vi "Variant to JSON.vi"(7 "Treatment of Infinity/NaN":T1, 8 "error in (no error)":errorcluster, 10 "Variant":variant) -> (0 "error out":errorcluster, 3 "JSON Value out":refnum<class "JSON Value.lvclass">)   [LabVIEW 2011, in "Variant JSON.lvlib"]
doc: "Converts a LabVIEW datatype (<b>Variant</b>) into a JSON value. Clusters are converted to JSON Objects. Variants, if empty (void), are converted to null, unless they have attributes, in which case these are converted into a JSON object. \n\nTreatment of Infinity, -Infinity, and Not-a-Number values of floating-point numerics:\n<b>-- Default JSON:</b> write all as nulls.\n<b>-- Extended:</b> use JSON strings for Infinities (\"Infinity\", \"-Infinity\"); NaN still null.\n<b>-- LabVIEW extentions</b> (compatable with the LabVIEW JSON primatives): Infinity, -Infinity, NaN (not in quotes)\n\nNote that the LabVIEW extentions are not valid JSON. The Extended option <b>is</b> valid JSON, but not all JSON parsers will process strings as numeric values.\n\nMore information on http://lavag.org/topic/16217-cr-json-labview"
uses:
  Variant JSON.lvlib
  JSON Value/JSON Value.lvclass
  JSON Scalar/Infinity&NaN.ctl
  <vilib>/Utility/VariantDataType/Type.ctl
  JSON Object/JSON Object.lvclass
  JSON Array/JSON Array.lvclass
  JSON Array/JSON Array.lvclass/JSON Array.ctl
  JSON Value/Set from JSON string.vi
  JSON Scalar/Set Null.vi
  JSON Scalar/Set I32.vi
  JSON Scalar/Set I64.vi
  JSON Scalar/Set U32.vi
  JSON Scalar/Set U64.vi
  JSON Scalar/Set SGL.vi
  JSON Scalar/Set EXT.vi
  JSON Scalar/Set Boolean.vi
  JSON Scalar/Set Path.vi
  JSON Scalar/Set Timestamp.vi
  JSON Scalar/JSON Scalar.lvclass
  Get Polymorphic/JSON GetSet.lvlib
  <vilib>/Utility/VariantDataType/VariantType.lvlib
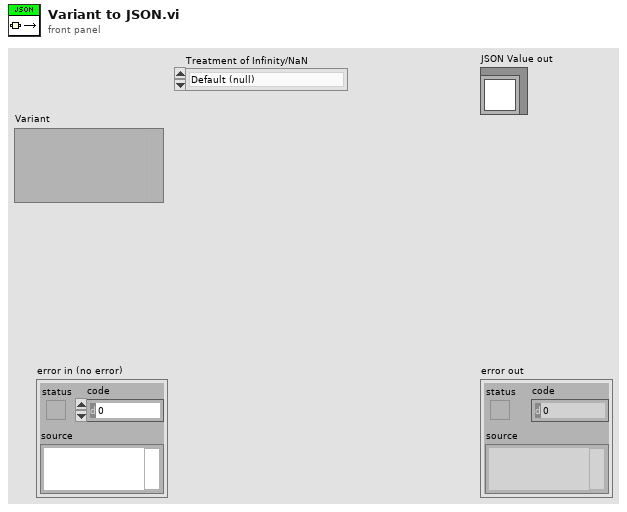
[diagram p1: front panel]
types:
  T1 = typedef "JSON Scalar.lvclass/Infinity&NaN.ctl" = enum16{"Default (null)", "Extended", "LabVIEW extensions"}
  T2 = typedef "VariantType.lvlib/Type.ctl" = enum8{"Invalid Type", "Void", "I8", "I16", "I32", "I64", "U8", "U16", "U32", "U64", "Single Float", "Double Float", "Extended Float", "Single Complex", "Double Complex", "Extended Complex", "Enum U8", "Enum U16", "Enum U32", "Enum U64", "Single Float With Unit", "Double Float With Unit", "Extended Float With Unit", "Single Complex with Unit", "Double Complex with Unit", "Extended Complex with Unit", "Boolean", "String", "Path", "Picture", "Tag", "Array", "Cluster", "Variant", "LV Variant", "Waveform", "Timestamp", "Digital Waveform", "Digital Data", "ExpressData", "Refnum", "External Data", "VI", "Poly VI", "LabVIEW Class Instance", "Fixed Point"}
  T3 = typedef "JSON Scalar.lvclass/Variant Data Typdef.ctl" = cluster{"Type Enum":T2, "Name":string, "Variant":variant}
  T4 = typedef "VariantType.lvlib/RefnumType.ctl" = enum16{"NotARefnum", "UnknownRefnum", "Generic", "Datalog", "ByteStream", "Device", "Occurence", "TCPNetConnection", "Auto", "Menu", "Imaq", "Hardware", "DataSocket", "Visa", "IVI", "UDPNetConnection", "Notifier", "Queue", "Irda", "EventReg", "DotNet", "UserEvent", "Callback", "UNUSED_EMPTY_POSITION", "BlueToothNetConnection", "LVObjApp", "LVObjVI", "LVObjUnknown", "GenericClass", "UserDefinedRefnumTag", "DataValue"}
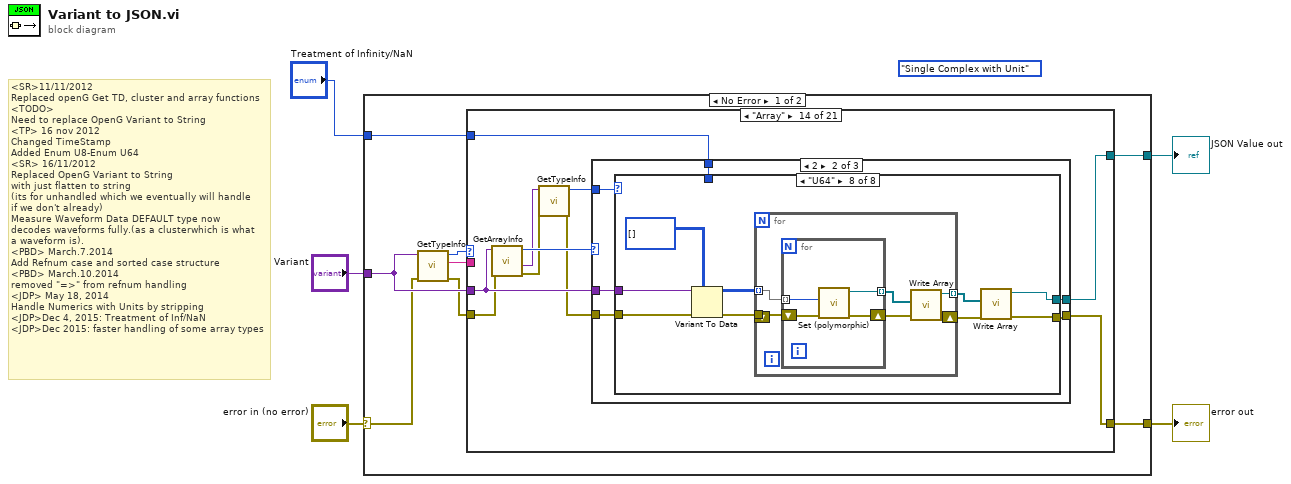
[diagram p0: block diagram]
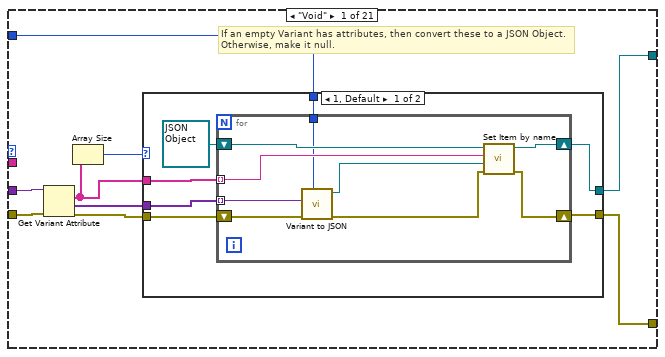
[diagram p2: hidden frame]
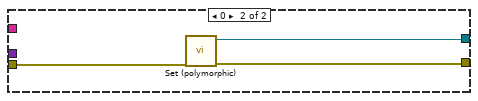
[diagram p3: hidden frame]
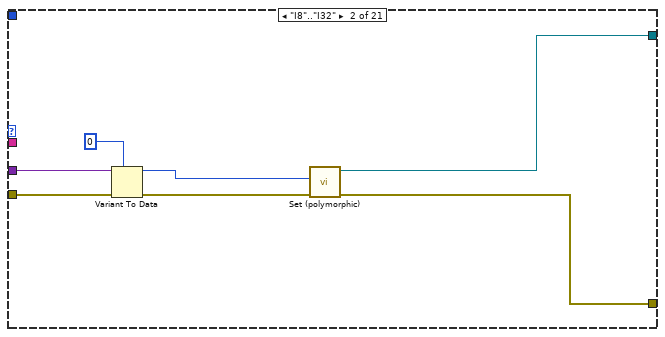
[diagram p4: hidden frame]
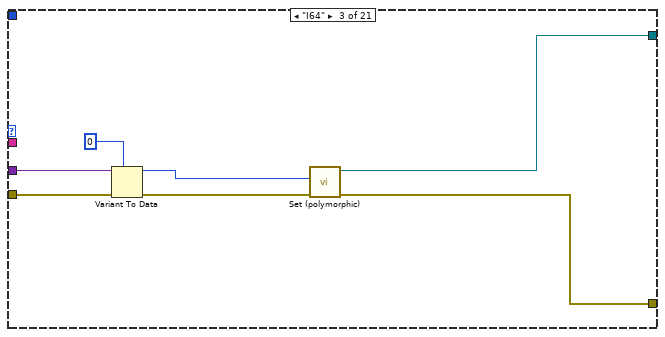
[diagram p5: hidden frame]
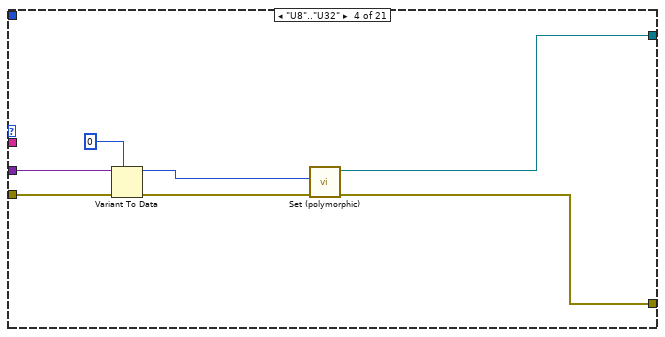
[diagram p6: hidden frame]
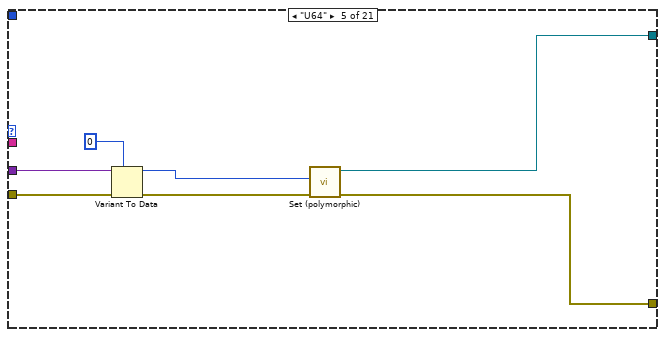
[diagram p7: hidden frame]
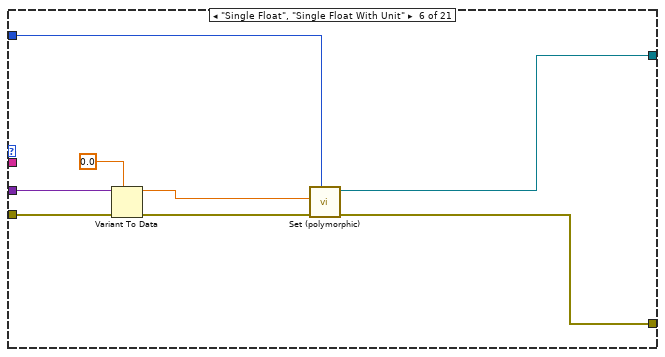
[diagram p8: hidden frame]
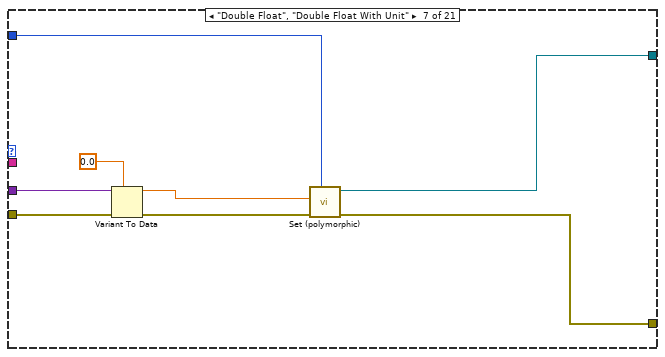
[diagram p9: hidden frame]
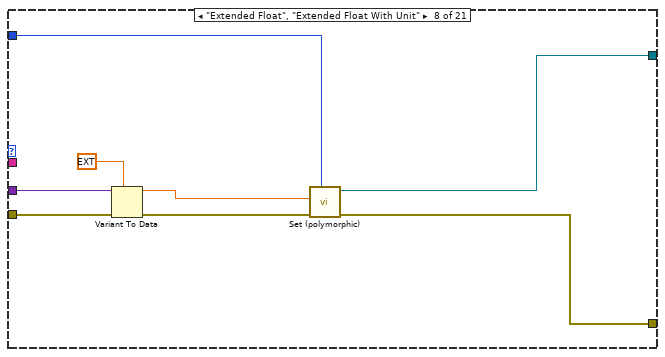
[diagram p10: hidden frame]
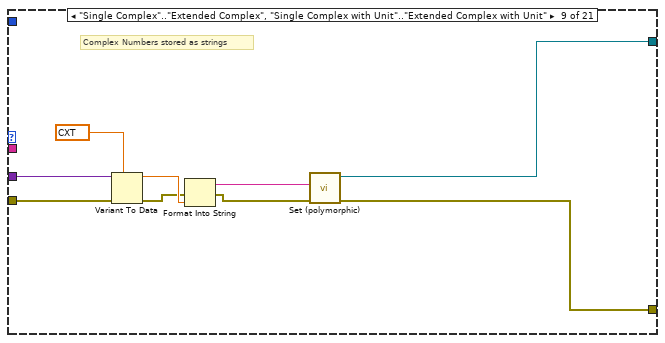
[diagram p11: hidden frame]
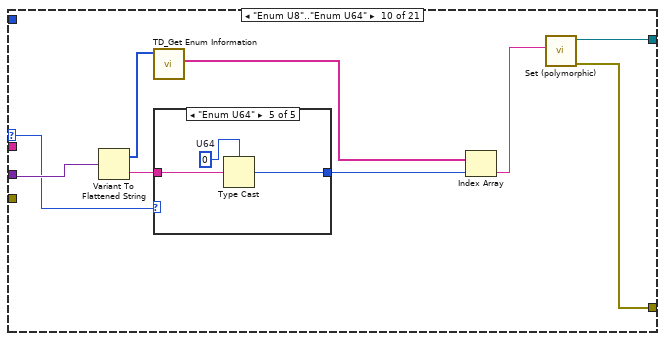
[diagram p12: hidden frame]
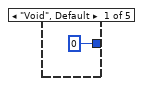
[diagram p13: hidden frame]
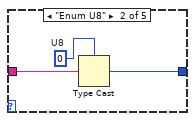
[diagram p14: hidden frame]
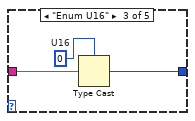
[diagram p15: hidden frame]
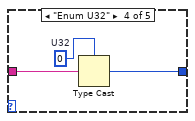
[diagram p16: hidden frame]
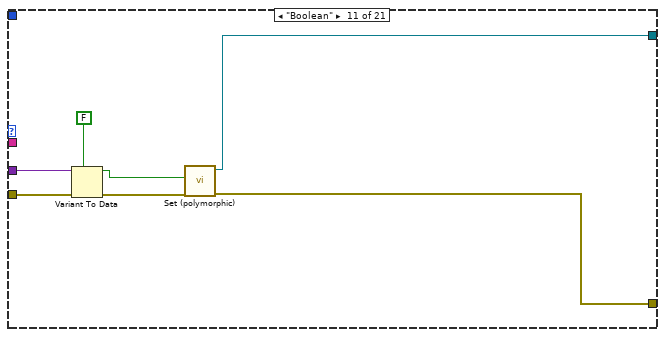
[diagram p17: hidden frame]
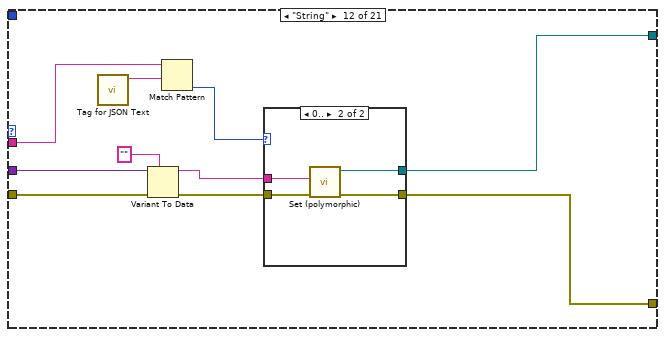
[diagram p18: hidden frame]
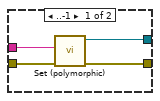
[diagram p19: hidden frame]
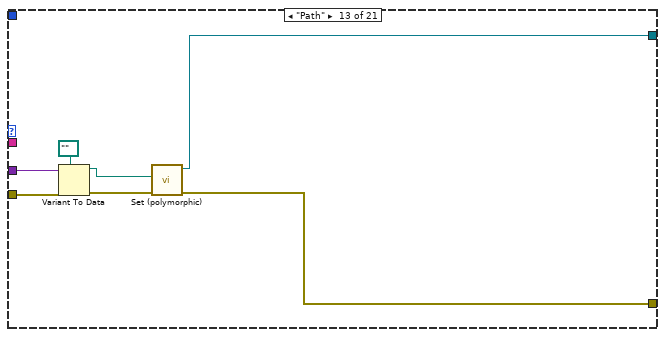
[diagram p20: hidden frame]
diagram:
  (unwired) Type."Single Complex with Unit" ("Type Enum")
  # "<SR>11/11/2012\nReplaced openG Get TD, cluster and array functions\n<TODO>\nNeed to replace OpenG Variant to String\n<TP> 16 nov 2012\nChanged TimeStamp\nAdded Enum U8-Enum U64\n<SR> 16/11/2012\nReplaced OpenG Variant to String\nwith just flatten to string \n(its for unhandled which we eventually will handle\nif we don't already)\nMeasure Waveform Data DEFAULT type now \ndecodes waveforms fully.(as a clusterwhich is what\na waveform is).\n<PBD> March.7.2014\nAdd Refnum case and sorted case structure\n<PBD> March.10.2014\nremoved \"=>\" from refnum handling\n<JDP> May 18, 2014\nHandle Numerics with Units by stripping\n<JDP>Dec 4, 2015: Treatment of Inf/NaN\n<JDP>Dec 2015: faster handling of some array types"
  n1 = case shown="No Error" "error in (no error)" {
    selector: "error in (no error)" -> [w10 w596]
    tunnel: [w12 w596] -> w4
    tunnel: [w13 _] -> w3
    tunnel: "Variant" -> [w11 _]
    tunnel: "Treatment of Infinity/NaN" -> [w6 _]
    frame No Error {
      n2 = call <vilib>:"GetTypeInfo.vi"("error in (no error)"=w10, "Variant"=w11) -> ("error out"=w9:errorcluster, "Name"=w7:string, "Type Enum"=w8:T2)  [unwired: 5 in, 2 out]
      n3 = case shown="\"Array\"" w8 {
        selector: w8 -> [_ _ _ _ _ _ _ _ _ w104 _ _ _ _ _ _ _ _ _ _ _]
        tunnel: w11 -> [w20 w48 w55 w62 w69 w77 w85 w93 w102 w105 w131 w141 w156 w163 w508 w526 w537 w544 w550 w580 w592]
        tunnel: [w22 w45 w52 w59 w66 w74 w82 w90 w101 w111 w128 w138 w152 w165 w511 w531 w539 w546 w548 w574 w595] -> w13
        tunnel: [w21 w43 w50 w57 w64 w72 w80 w88 w100 w110 w126 w136 w151 w166 w510 w530 w538 w545 w547 w573 w594] -> w12
        tunnel: w9 -> [w15 w42 w49 w56 w63 w71 w79 w87 w99 _ w125 w135 w154 w162 w506 w525 w536 w540 w549 w579 w593]
        tunnel: w7 -> [_ _ _ _ _ _ _ _ _ _ _ w133 _ _ _ _ _ _ _ _ _]
        tunnel: w6 -> [w14 _ _ _ _ w70 w78 w86 _ _ _ _ _ w164 w505 w524 w535 _ _ _ _]
        frame "Void" {
          # "If an empty Variant has attributes, then convert these to a JSON Object.\nOtherwise, make it null."
          n4 = Get Variant Attribute(Variant=w20, error in=w15) -> (names=w18:string[], values=w17:variant[], error out=w16:errorcluster)  [unwired: 2 in, 1 out]
          n5 = Array Size(array=w18) -> (size(s)=w19:i32)
          n6 = case shown="1, Default" w19 {
            tunnel: [w25 w40] -> w21
            tunnel: [w24 w41] -> w22
            tunnel: w18 -> [w27 _]
            tunnel: w17 -> [w29 _]
            tunnel: w16 -> [w28 w39]
            tunnel: w14 -> [w23 _]
            frame 1, Default {
              n7 = for {
                tunnel: w29 -> [w35] mode=indexing
                shift-right: [w31] -> w25
                shift-left: w28 -> [w34]
                tunnel: w27 -> [w36] mode=indexing
                shift-right: [w38] -> w24
                shift-left: refnum<class "JSON Object.lvclass"> refnum ("JSON Object out") -> [w37]
                tunnel: w23 -> [w30]
                n8 = call "Variant to JSON.vi"("Treatment of Infinity/NaN"=w30, "error in (no error)"=w34, "Variant"=w35) -> ("error out"=w32:errorcluster, "JSON Value out"=w33:refnum<class "JSON Value.lvclass">)  [unwired: 7 in]
                n9 = call-dynamic "Set Item by name.vi"("error in (no error)"=w32, "Value"=w33, "name"=w36, "JSON Object in"=w37) -> ("error out"=w31:errorcluster, "JSON Object out"=w38:refnum<class "JSON Object.lvclass">)  [unwired: 5 in, 1 out]
              }
            }
            frame 0 {
              n10 = call-poly "Set (polymorphic).vi"("error in (no error)"=w39) -> ("error out"=w40:errorcluster, "JSON Scalar out"=w41:refnum<class "JSON Scalar.lvclass">)  [unwired: 9 in]
            }
          }
        }
        frame "I8".."I32" {
          n11 = Variant To Data(error in=w42, type=0, Variant=w48) -> (data=w46:i32, error out=w44:errorcluster)
          n12 = call-poly "Set (polymorphic).vi"("error in (no error)"=w44, "Numeric"=w46) -> ("error out"=w43:errorcluster, "JSON Scalar out"=w45:refnum<class "JSON Scalar.lvclass">)  [unwired: 8 in]
        }
        frame "I64" {
          n13 = Variant To Data(error in=w49, type=i64 0, Variant=w55) -> (data=w53:i64, error out=w51:errorcluster)
          n14 = call-poly "Set (polymorphic).vi"("error in (no error)"=w51, "Numeric"=w53) -> ("error out"=w50:errorcluster, "JSON Scalar out"=w52:refnum<class "JSON Scalar.lvclass">)  [unwired: 8 in]
        }
        frame "U8".."U32" {
          n15 = Variant To Data(error in=w56, type=u32 0, Variant=w62) -> (data=w60:u32, error out=w58:errorcluster)
          n16 = call-poly "Set (polymorphic).vi"("error in (no error)"=w58, "Numeric"=w60) -> ("error out"=w57:errorcluster, "JSON Scalar out"=w59:refnum<class "JSON Scalar.lvclass">)  [unwired: 8 in]
        }
        frame "U64" {
          n17 = Variant To Data(error in=w63, type=u64 0, Variant=w69) -> (data=w67:u64, error out=w65:errorcluster)
          n18 = call-poly "Set (polymorphic).vi"("error in (no error)"=w65, "Numeric"=w67) -> ("error out"=w64:errorcluster, "JSON Scalar out"=w66:refnum<class "JSON Scalar.lvclass">)  [unwired: 8 in]
        }
        frame "Single Float", "Single Float With Unit" {
          n19 = Variant To Data(error in=w71, type=sgl 0.0, Variant=w77) -> (data=w75:sgl, error out=w73:errorcluster)
          n20 = call-poly "Set (polymorphic).vi"("Treatment of Infinity/NaN"=w70, "error in (no error)"=w73, "Numeric"=w75) -> ("error out"=w72:errorcluster, "JSON Scalar out"=w74:refnum<class "JSON Scalar.lvclass">)  [unwired: 7 in]
        }
        frame "Double Float", "Double Float With Unit" {
          n21 = Variant To Data(error in=w79, type=0.0, Variant=w85) -> (data=w83:dbl, error out=w81:errorcluster)
          n22 = call-poly "Set (polymorphic).vi"("Treatment of Infinity/NaN"=w78, "error in (no error)"=w81, "Numeric"=w83) -> ("error out"=w80:errorcluster, "JSON Scalar out"=w82:refnum<class "JSON Scalar.lvclass">)  [unwired: 7 in]
        }
        frame "Extended Float", "Extended Float With Unit" {
          n23 = Variant To Data(error in=w87, type=ext 0.0, Variant=w93) -> (data=w91:ext, error out=w89:errorcluster)
          n24 = call-poly "Set (polymorphic).vi"("Treatment of Infinity/NaN"=w86, "error in (no error)"=w89, "Numeric"=w91) -> ("error out"=w88:errorcluster, "JSON Scalar out"=w90:refnum<class "JSON Scalar.lvclass">)  [unwired: 7 in]
        }
        frame "Single Complex".."Extended Complex", "Single Complex with Unit".."Extended Complex with Unit" {
          # "Complex Numbers stored as strings"
          n25 = Variant To Data(error in=w99, type=cxt 0.0+0.0i, Variant=w102) -> (data=w97:cxt, error out=w95:errorcluster)
          n26 = Format Into String(error in=w95, w97) -> (resulting string=w96:string, error out=w94:errorcluster)  [unwired: 2 in]
          n27 = call-poly "Set (polymorphic).vi"("error in (no error)"=w94, "String"=w96) -> ("error out"=w100:errorcluster, "JSON Scalar out"=w101:refnum<class "JSON Scalar.lvclass">)  [unwired: 8 in]
        }
        frame "Enum U8".."Enum U64" {
          n28 = Variant To Flattened String(Variant=w105) -> (data string=w108:string, 1:w109:i16[])
          n29 = call <vilib>:"TD_Get Enum Information.vi"("Type descriptor"=w109) -> ("Value Names"=w107:string[])  [unwired: 9 in, 1 out]
          n30 = case shown="\"Enum U64\"" w104 {
            tunnel: w108 -> [_ w115 w118 w121 w124]
            tunnel: [u64 0 ("U8") w113 w116 w119 w122] -> w106
            frame "Void", Default {
            }
            frame "Enum U8" {
              w114 = u8 0  # U8
              n31 = Type Cast(type=w114, x=w115) -> (*(type *) &x=w113:u8)
            }
            frame "Enum U16" {
              w117 = u16 0  # U16
              n32 = Type Cast(type=w117, x=w118) -> (*(type *) &x=w116:u16)
            }
            frame "Enum U32" {
              w120 = u32 0  # U32
              n33 = Type Cast(type=w120, x=w121) -> (*(type *) &x=w119:u32)
            }
            frame "Enum U64" {
              w123 = u64 0  # U64
              n34 = Type Cast(type=w123, x=w124) -> (*(type *) &x=w122:u64)
            }
          }
          n35 = Index Array(array=w107, index=w106) -> (element=w103:string)
          n36 = call-poly "Set (polymorphic).vi"("String"=w103) -> ("error out"=w110:errorcluster, "JSON Scalar out"=w111:refnum<class "JSON Scalar.lvclass">)  [unwired: 9 in]
        }
        frame "Boolean" {
          n37 = Variant To Data(error in=w125, type=FALSE, Variant=w131) -> (data=w129:bool, error out=w127:errorcluster)
          n38 = call-poly "Set (polymorphic).vi"("error in (no error)"=w127, "Boolean"=w129) -> ("error out"=w126:errorcluster, "JSON Scalar out"=w128:refnum<class "JSON Scalar.lvclass">)  [unwired: 8 in]
        }
        frame "String" {
          n39 = call "Tag for JSON Text.vi"() -> ("Tag for JSON text"=w134:string)  [unwired: 11 in]
          n40 = Variant To Data(error in=w135, type="", Variant=w141) -> (data=w139:string, error out=w137:errorcluster)
          n41 = Match Pattern(string=w133, regular expression=w134) -> (offset past match=w132:i32)  [unwired: 1 in, 3 out]
          n42 = case shown="0.." w132 {
            tunnel: w139 -> [w145 w149]
            tunnel: [w144 w148] -> w138
            tunnel: w137 -> [w143 w147]
            tunnel: [w142 w146] -> w136
            frame ..-1 {
              n43 = call-poly "Set (polymorphic).vi"("error in (no error)"=w143, "String"=w145) -> ("error out"=w142:errorcluster, "JSON Scalar out"=w144:refnum<class "JSON Scalar.lvclass">)  [unwired: 8 in]
            }
            frame 0.. {
              n44 = call-poly "Set (polymorphic).vi"("error in (no error)"=w147, "JSON stream"=w149) -> ("error out"=w146:errorcluster, "JSON Value out"=w148:refnum<class "JSON Value.lvclass">)  [unwired: 7 in, 1 out]
            }
          }
        }
        frame "Path" {
          n45 = Variant To Data(error in=w154, type=path "", Variant=w156) -> (data=w150:path, error out=w153:errorcluster)
          n46 = call-poly "Set (polymorphic).vi"("error in (no error)"=w153, "Path"=w150) -> ("error out"=w151:errorcluster, "JSON Scalar out"=w152:refnum<class "JSON Scalar.lvclass">)  [unwired: 8 in]
        }
        frame "Array" {
          n47 = call <vilib>:"GetArrayInfo.vi"("error in (no error)"=w162, "Variant"=w163) -> ("error out"=w160:errorcluster, "ArrayElement"=w159:variant, "NDims"=w161:i32)  [unwired: 6 in, 1 out]
          n48 = call <vilib>:"GetTypeInfo.vi"("error in (no error)"=w160, "Variant"=w159) -> ("error out"=w158:errorcluster, "Type Enum"=w157:T2)  [unwired: 5 in, 3 out]
          n49 = case shown="2" w161 {
            tunnel: [w171 w331 w504] -> w166
            tunnel: [w170 w330 w500] -> w165
            tunnel: w164 -> [w168 w328 w499]
            tunnel: w163 -> [w172 w332 w498]
            tunnel: w158 -> [w169 w329 w497]
            tunnel: w157 -> [w167 w327 _]
            frame 1 {
              n50 = case shown="\"Waveform\"" w167 {
                tunnel: w172 -> [w183 w197 w211 w226 w241 w255 w268 w281 w294 w307 w321]
                tunnel: [w177 w191 w205 w220 w235 w249 w262 w275 w288 w301 w315] -> w171
                tunnel: [w176 w190 w204 w219 w234 w248 w261 w274 w287 w300 w314] -> w170
                tunnel: w169 -> [w174 w189 w203 w218 w233 w247 w260 w273 w286 w299 w313]
                tunnel: w168 -> [w173 _ w202 w217 w232 _ _ _ _ _ w312]
                frame Default {
                  n51 = Variant To Data(error in=w174, type=variant[] [], Variant=w183) -> (data=w181:variant[], error out=w180:errorcluster)
                  n52 = for {
                    tunnel: w181 -> [w188] mode=indexing
                    shift-right: [w186] -> w178
                    shift-left: w180 -> [w187]
                    tunnel: [w185] -> w179 mode=indexing
                    tunnel: w173 -> [w184]
                    n53 = call "Variant to JSON.vi"("Treatment of Infinity/NaN"=w184, "error in (no error)"=w187, "Variant"=w188) -> ("error out"=w186:errorcluster, "JSON Value out"=w185:refnum<class "JSON Value.lvclass">)  [unwired: 7 in]
                  }
                  n54 = call "Write Array.vi"("error in (no error)"=w178, "Array"=w179, "JSON Array in"=refnum<class "JSON Array.lvclass"> refnum) -> ("error out"=w177:errorcluster, "JSON Array out"=w176:refnum<class "JSON Array.lvclass">)  [unwired: 7 in]
                }
                frame "String" {
                  n55 = Variant To Data(error in=w189, type=string[] [], Variant=w197) -> (data=w195:string[], error out=w194:errorcluster)
                  n56 = for {
                    tunnel: w195 -> [w198] mode=indexing
                    shift-right: [w200] -> w192
                    shift-left: w194 -> [w201]
                    tunnel: [w199] -> w193 mode=indexing
                    n57 = call "Set String.vi"("error in (no error)"=w201, "String"=w198) -> ("error out"=w200:errorcluster, "JSON Scalar out"=w199:refnum<class "JSON Scalar.lvclass">)  [unwired: 8 in]
                  }
                  n58 = call "Write Array.vi"("error in (no error)"=w192, "Array"=w193) -> ("error out"=w191:errorcluster, "JSON Array out"=w190:refnum<class "JSON Array.lvclass">)  [unwired: 8 in]
                }
                frame "Single Float" {
                  n59 = Variant To Data(error in=w203, type=sgl[] [], Variant=w211) -> (data=w209:sgl[], error out=w208:errorcluster)
                  n60 = for {
                    tunnel: w209 -> [w212] mode=indexing
                    shift-right: [w215] -> w206
                    shift-left: w208 -> [w216]
                    tunnel: [w214] -> w207 mode=indexing
                    tunnel: w202 -> [w213]
                    n61 = call "Set DBL.vi"("Treatment of Infinity/NaN"=w213, "error in (no error)"=w216, "Numeric"=w212) -> ("error out"=w215:errorcluster, "JSON Scalar out"=w214:refnum<class "JSON Scalar.lvclass">)  [unwired: 7 in]
                  }
                  n62 = call "Write Array.vi"("error in (no error)"=w206, "Array"=w207) -> ("error out"=w205:errorcluster, "JSON Array out"=w204:refnum<class "JSON Array.lvclass">)  [unwired: 8 in]
                }
                frame "Double Float" {
                  n63 = Variant To Data(error in=w218, type=dbl[] [], Variant=w226) -> (data=w224:dbl[], error out=w223:errorcluster)
                  n64 = for {
                    tunnel: w224 -> [w227] mode=indexing
                    shift-right: [w230] -> w221
                    shift-left: w223 -> [w231]
                    tunnel: [w229] -> w222 mode=indexing
                    tunnel: w217 -> [w228]
                    n65 = call-poly "Set (polymorphic).vi"("Treatment of Infinity/NaN"=w228, "error in (no error)"=w231, "Numeric"=w227) -> ("error out"=w230:errorcluster, "JSON Scalar out"=w229:refnum<class "JSON Scalar.lvclass">)  [unwired: 7 in]
                  }
                  n66 = call "Write Array.vi"("error in (no error)"=w221, "Array"=w222) -> ("error out"=w220:errorcluster, "JSON Array out"=w219:refnum<class "JSON Array.lvclass">)  [unwired: 8 in]
                }
                frame "Extended Float" {
                  n67 = Variant To Data(error in=w233, type=ext[] [], Variant=w241) -> (data=w239:ext[], error out=w238:errorcluster)
                  n68 = for {
                    tunnel: w239 -> [w242] mode=indexing
                    shift-right: [w245] -> w236
                    shift-left: w238 -> [w246]
                    tunnel: [w244] -> w237 mode=indexing
                    tunnel: w232 -> [w243]
                    n69 = call-poly "Set (polymorphic).vi"("Treatment of Infinity/NaN"=w243, "error in (no error)"=w246, "Numeric"=w242) -> ("error out"=w245:errorcluster, "JSON Scalar out"=w244:refnum<class "JSON Scalar.lvclass">)  [unwired: 7 in]
                  }
                  n70 = call "Write Array.vi"("error in (no error)"=w236, "Array"=w237) -> ("error out"=w235:errorcluster, "JSON Array out"=w234:refnum<class "JSON Array.lvclass">)  [unwired: 8 in]
                }
                frame "I8".."I32" {
                  n71 = Variant To Data(error in=w247, type=i32[] [], Variant=w255) -> (data=w253:i32[], error out=w252:errorcluster)
                  n72 = for {
                    tunnel: w253 -> [w256] mode=indexing
                    shift-right: [w258] -> w250
                    shift-left: w252 -> [w259]
                    tunnel: [w257] -> w251 mode=indexing
                    n73 = call-poly "Set (polymorphic).vi"("error in (no error)"=w259, "Numeric"=w256) -> ("error out"=w258:errorcluster, "JSON Scalar out"=w257:refnum<class "JSON Scalar.lvclass">)  [unwired: 8 in]
                  }
                  n74 = call "Write Array.vi"("error in (no error)"=w250, "Array"=w251) -> ("error out"=w249:errorcluster, "JSON Array out"=w248:refnum<class "JSON Array.lvclass">)  [unwired: 8 in]
                }
                frame "I64" {
                  n75 = Variant To Data(error in=w260, type=i64[] [], Variant=w268) -> (data=w266:i64[], error out=w265:errorcluster)
                  n76 = for {
                    tunnel: w266 -> [w269] mode=indexing
                    shift-right: [w271] -> w263
                    shift-left: w265 -> [w272]
                    tunnel: [w270] -> w264 mode=indexing
                    n77 = call-poly "Set (polymorphic).vi"("error in (no error)"=w272, "Numeric"=w269) -> ("error out"=w271:errorcluster, "JSON Scalar out"=w270:refnum<class "JSON Scalar.lvclass">)  [unwired: 8 in]
                  }
                  n78 = call "Write Array.vi"("error in (no error)"=w263, "Array"=w264) -> ("error out"=w262:errorcluster, "JSON Array out"=w261:refnum<class "JSON Array.lvclass">)  [unwired: 8 in]
                }
                frame "U8".."U32" {
                  n79 = Variant To Data(error in=w273, type=u32[] [], Variant=w281) -> (data=w279:u32[], error out=w278:errorcluster)
                  n80 = for {
                    tunnel: w279 -> [w282] mode=indexing
                    shift-right: [w284] -> w276
                    shift-left: w278 -> [w285]
                    tunnel: [w283] -> w277 mode=indexing
                    n81 = call-poly "Set (polymorphic).vi"("error in (no error)"=w285, "Numeric"=w282) -> ("error out"=w284:errorcluster, "JSON Scalar out"=w283:refnum<class "JSON Scalar.lvclass">)  [unwired: 8 in]
                  }
                  n82 = call "Write Array.vi"("error in (no error)"=w276, "Array"=w277) -> ("error out"=w275:errorcluster, "JSON Array out"=w274:refnum<class "JSON Array.lvclass">)  [unwired: 8 in]
                }
                frame "U64" {
                  n83 = Variant To Data(error in=w286, type=u64[] [], Variant=w294) -> (data=w292:u64[], error out=w291:errorcluster)
                  n84 = for {
                    tunnel: w292 -> [w295] mode=indexing
                    shift-right: [w297] -> w289
                    shift-left: w291 -> [w298]
                    tunnel: [w296] -> w290 mode=indexing
                    n85 = call-poly "Set (polymorphic).vi"("error in (no error)"=w298, "Numeric"=w295) -> ("error out"=w297:errorcluster, "JSON Scalar out"=w296:refnum<class "JSON Scalar.lvclass">)  [unwired: 8 in]
                  }
                  n86 = call "Write Array.vi"("error in (no error)"=w289, "Array"=w290) -> ("error out"=w288:errorcluster, "JSON Array out"=w287:refnum<class "JSON Array.lvclass">)  [unwired: 8 in]
                }
                frame "Timestamp" {
                  n87 = Variant To Data(error in=w299, type=timestamp[] [], Variant=w307) -> (data=w305:timestamp[], error out=w304:errorcluster)
                  n88 = for {
                    tunnel: w305 -> [w308] mode=indexing
                    shift-right: [w310] -> w302
                    shift-left: w304 -> [w311]
                    tunnel: [w309] -> w303 mode=indexing
                    n89 = call-poly "Set (polymorphic).vi"("error in (no error)"=w311, "Time Stamp"=w308) -> ("error out"=w310:errorcluster, "JSON Scalar out"=w309:refnum<class "JSON Scalar.lvclass">)  [unwired: 8 in]
                  }
                  n90 = call "Write Array.vi"("error in (no error)"=w302, "Array"=w303) -> ("error out"=w301:errorcluster, "JSON Array out"=w300:refnum<class "JSON Array.lvclass">)  [unwired: 8 in]
                }
                frame "Waveform" {
                  n91 = Variant To Data(error in=w313, type=waveform(dbl)[] [], Variant=w321) -> (data=w319:waveform(dbl)[], error out=w318:errorcluster)
                  n92 = for {
                    tunnel: w319 -> [w323] mode=indexing
                    shift-right: [w325] -> w316
                    shift-left: w318 -> [w326]
                    tunnel: [w324] -> w317 mode=indexing
                    tunnel: w312 -> [w322]
                    n93 = call-poly "Set (polymorphic).vi"("Treatment of Infinity/NaN"=w322, "error in (no error)"=w326, "waveform"=w323) -> ("error out"=w325:errorcluster, "JSON Object out"=w324:refnum<class "JSON Object.lvclass">)  [unwired: 7 in]
                  }
                  n94 = call "Write Array.vi"("error in (no error)"=w316, "Array"=w317) -> ("error out"=w315:errorcluster, "JSON Array out"=w314:refnum<class "JSON Array.lvclass">)  [unwired: 8 in]
                }
              }
            }
            frame 2 {
              n95 = case shown="\"U64\"" w327 {
                tunnel: w332 -> [w342 w364 w386 w408 w429 w448 w467 w486]
                tunnel: [w334 w356 w378 w400 w422 w441 w460 w479] -> w331
                tunnel: [w333 w355 w377 w399 w421 w440 w459 w478] -> w330
                tunnel: w329 -> [w338 w360 w382 w404 w425 w444 w463 w482]
                tunnel: w328 -> [w337 w359 w381 w403 _ _ _ _]
                frame Default {
                  n96 = Variant To Data(error in=w338, type=variant[][] [], Variant=w342) -> (data=w340:variant[][], error out=w339:errorcluster)
                  n97 = for {
                    tunnel: w340 -> [w349] mode=indexing
                    tunnel: w339 -> [w348]
                    tunnel: [w344] -> w336 mode=indexing
                    tunnel: w337 -> [w343]
                    shift-right: [w345] -> w335
                    shift-left: _ -> [_]
                    n98 = for {
                      tunnel: w349 -> [w354] mode=indexing
                      shift-right: [w352] -> w346
                      shift-left: w348 -> [w353]
                      tunnel: [w351] -> w347 mode=indexing
                      tunnel: w343 -> [w350]
                      n99 = call "Variant to JSON.vi"("Treatment of Infinity/NaN"=w350, "error in (no error)"=w353, "Variant"=w354) -> ("error out"=w352:errorcluster, "JSON Value out"=w351:refnum<class "JSON Value.lvclass">)  [unwired: 7 in]
                    }
                    n100 = call "Write Array.vi"("error in (no error)"=w346, "Array"=w347) -> ("error out"=w345:errorcluster, "JSON Array out"=w344:refnum<class "JSON Array.lvclass">)  [unwired: 8 in]
                  }
                  n101 = call "Write Array.vi"("error in (no error)"=w335, "Array"=w336) -> ("error out"=w334:errorcluster, "JSON Array out"=w333:refnum<class "JSON Array.lvclass">)  [unwired: 8 in]
                }
                frame "Double Float" {
                  n102 = Variant To Data(error in=w360, type=dbl[][] [], Variant=w364) -> (data=w362:dbl[][], error out=w361:errorcluster)
                  n103 = for {
                    tunnel: w362 -> [w371] mode=indexing
                    tunnel: w361 -> [w370]
                    tunnel: [w366] -> w358 mode=indexing
                    tunnel: w359 -> [w365]
                    shift-right: [w367] -> w357
                    shift-left: _ -> [_]
                    n104 = for {
                      tunnel: w371 -> [w372] mode=indexing
                      shift-right: [w375] -> w368
                      shift-left: w370 -> [w376]
                      tunnel: [w374] -> w369 mode=indexing
                      tunnel: w365 -> [w373]
                      n105 = call "Set DBL.vi"("Treatment of Infinity/NaN"=w373, "error in (no error)"=w376, "Numeric"=w372) -> ("error out"=w375:errorcluster, "JSON Scalar out"=w374:refnum<class "JSON Scalar.lvclass">)  [unwired: 7 in]
                    }
                    n106 = call "Write Array.vi"("error in (no error)"=w368, "Array"=w369) -> ("error out"=w367:errorcluster, "JSON Array out"=w366:refnum<class "JSON Array.lvclass">)  [unwired: 8 in]
                  }
                  n107 = call "Write Array.vi"("error in (no error)"=w357, "Array"=w358) -> ("error out"=w356:errorcluster, "JSON Array out"=w355:refnum<class "JSON Array.lvclass">)  [unwired: 8 in]
                }
                frame "Single Float" {
                  n108 = Variant To Data(error in=w382, type=sgl[][] [], Variant=w386) -> (data=w384:sgl[][], error out=w383:errorcluster)
                  n109 = for {
                    tunnel: w384 -> [w393] mode=indexing
                    tunnel: w383 -> [w392]
                    tunnel: [w388] -> w380 mode=indexing
                    tunnel: w381 -> [w387]
                    shift-right: [w389] -> w379
                    shift-left: _ -> [_]
                    n110 = for {
                      tunnel: w393 -> [w394] mode=indexing
                      shift-right: [w397] -> w390
                      shift-left: w392 -> [w398]
                      tunnel: [w396] -> w391 mode=indexing
                      tunnel: w387 -> [w395]
                      n111 = call-poly "Set (polymorphic).vi"("Treatment of Infinity/NaN"=w395, "error in (no error)"=w398, "Numeric"=w394) -> ("error out"=w397:errorcluster, "JSON Scalar out"=w396:refnum<class "JSON Scalar.lvclass">)  [unwired: 7 in]
                    }
                    n112 = call "Write Array.vi"("error in (no error)"=w390, "Array"=w391) -> ("error out"=w389:errorcluster, "JSON Array out"=w388:refnum<class "JSON Array.lvclass">)  [unwired: 8 in]
                  }
                  n113 = call "Write Array.vi"("error in (no error)"=w379, "Array"=w380) -> ("error out"=w378:errorcluster, "JSON Array out"=w377:refnum<class "JSON Array.lvclass">)  [unwired: 8 in]
                }
                frame "Extended Float" {
                  n114 = Variant To Data(error in=w404, type=ext[][] [], Variant=w408) -> (data=w406:ext[][], error out=w405:errorcluster)
                  n115 = for {
                    tunnel: w406 -> [w415] mode=indexing
                    tunnel: w405 -> [w414]
                    tunnel: [w410] -> w402 mode=indexing
                    tunnel: w403 -> [w409]
                    shift-right: [w411] -> w401
                    shift-left: _ -> [_]
                    n116 = for {
                      tunnel: w415 -> [w416] mode=indexing
                      shift-right: [w419] -> w412
                      shift-left: w414 -> [w420]
                      tunnel: [w418] -> w413 mode=indexing
                      tunnel: w409 -> [w417]
                      n117 = call-poly "Set (polymorphic).vi"("Treatment of Infinity/NaN"=w417, "error in (no error)"=w420, "Numeric"=w416) -> ("error out"=w419:errorcluster, "JSON Scalar out"=w418:refnum<class "JSON Scalar.lvclass">)  [unwired: 7 in]
                    }
                    n118 = call "Write Array.vi"("error in (no error)"=w412, "Array"=w413) -> ("error out"=w411:errorcluster, "JSON Array out"=w410:refnum<class "JSON Array.lvclass">)  [unwired: 8 in]
                  }
                  n119 = call "Write Array.vi"("error in (no error)"=w401, "Array"=w402) -> ("error out"=w400:errorcluster, "JSON Array out"=w399:refnum<class "JSON Array.lvclass">)  [unwired: 8 in]
                }
                frame "I8".."I32" {
                  n120 = Variant To Data(error in=w425, type=i32[][] [], Variant=w429) -> (data=w427:i32[][], error out=w426:errorcluster)
                  n121 = for {
                    tunnel: w427 -> [w435] mode=indexing
                    tunnel: w426 -> [w434]
                    tunnel: [w430] -> w424 mode=indexing
                    shift-right: [w431] -> w423
                    shift-left: _ -> [_]
                    n122 = for {
                      tunnel: w435 -> [w436] mode=indexing
                      shift-right: [w438] -> w432
                      shift-left: w434 -> [w439]
                      tunnel: [w437] -> w433 mode=indexing
                      n123 = call-poly "Set (polymorphic).vi"("error in (no error)"=w439, "Numeric"=w436) -> ("error out"=w438:errorcluster, "JSON Scalar out"=w437:refnum<class "JSON Scalar.lvclass">)  [unwired: 8 in]
                    }
                    n124 = call "Write Array.vi"("error in (no error)"=w432, "Array"=w433) -> ("error out"=w431:errorcluster, "JSON Array out"=w430:refnum<class "JSON Array.lvclass">)  [unwired: 8 in]
                  }
                  n125 = call "Write Array.vi"("error in (no error)"=w423, "Array"=w424) -> ("error out"=w422:errorcluster, "JSON Array out"=w421:refnum<class "JSON Array.lvclass">)  [unwired: 8 in]
                }
                frame "I64" {
                  n126 = Variant To Data(error in=w444, type=i64[][] [], Variant=w448) -> (data=w446:i64[][], error out=w445:errorcluster)
                  n127 = for {
                    tunnel: w446 -> [w454] mode=indexing
                    tunnel: w445 -> [w453]
                    tunnel: [w449] -> w443 mode=indexing
                    shift-right: [w450] -> w442
                    shift-left: _ -> [_]
                    n128 = for {
                      tunnel: w454 -> [w455] mode=indexing
                      shift-right: [w457] -> w451
                      shift-left: w453 -> [w458]
                      tunnel: [w456] -> w452 mode=indexing
                      n129 = call-poly "Set (polymorphic).vi"("error in (no error)"=w458, "Numeric"=w455) -> ("error out"=w457:errorcluster, "JSON Scalar out"=w456:refnum<class "JSON Scalar.lvclass">)  [unwired: 8 in]
                    }
                    n130 = call "Write Array.vi"("error in (no error)"=w451, "Array"=w452) -> ("error out"=w450:errorcluster, "JSON Array out"=w449:refnum<class "JSON Array.lvclass">)  [unwired: 8 in]
                  }
                  n131 = call "Write Array.vi"("error in (no error)"=w442, "Array"=w443) -> ("error out"=w441:errorcluster, "JSON Array out"=w440:refnum<class "JSON Array.lvclass">)  [unwired: 8 in]
                }
                frame "U8".."U32" {
                  n132 = Variant To Data(error in=w463, type=u32[][] [], Variant=w467) -> (data=w465:u32[][], error out=w464:errorcluster)
                  n133 = for {
                    tunnel: w465 -> [w473] mode=indexing
                    tunnel: w464 -> [w472]
                    tunnel: [w468] -> w462 mode=indexing
                    shift-right: [w469] -> w461
                    shift-left: _ -> [_]
                    n134 = for {
                      tunnel: w473 -> [w474] mode=indexing
                      shift-right: [w476] -> w470
                      shift-left: w472 -> [w477]
                      tunnel: [w475] -> w471 mode=indexing
                      n135 = call-poly "Set (polymorphic).vi"("error in (no error)"=w477, "Numeric"=w474) -> ("error out"=w476:errorcluster, "JSON Scalar out"=w475:refnum<class "JSON Scalar.lvclass">)  [unwired: 8 in]
                    }
                    n136 = call "Write Array.vi"("error in (no error)"=w470, "Array"=w471) -> ("error out"=w469:errorcluster, "JSON Array out"=w468:refnum<class "JSON Array.lvclass">)  [unwired: 8 in]
                  }
                  n137 = call "Write Array.vi"("error in (no error)"=w461, "Array"=w462) -> ("error out"=w460:errorcluster, "JSON Array out"=w459:refnum<class "JSON Array.lvclass">)  [unwired: 8 in]
                }
                frame "U64" {
                  n138 = Variant To Data(error in=w482, type=u64[][] [], Variant=w486) -> (data=w484:u64[][], error out=w483:errorcluster)
                  n139 = for {
                    tunnel: w484 -> [w492] mode=indexing
                    tunnel: w483 -> [w491]
                    tunnel: [w487] -> w481 mode=indexing
                    shift-right: [w488] -> w480
                    shift-left: _ -> [_]
                    n140 = for {
                      tunnel: w492 -> [w493] mode=indexing
                      shift-right: [w495] -> w489
                      shift-left: w491 -> [w496]
                      tunnel: [w494] -> w490 mode=indexing
                      n141 = call-poly "Set (polymorphic).vi"("error in (no error)"=w496, "Numeric"=w493) -> ("error out"=w495:errorcluster, "JSON Scalar out"=w494:refnum<class "JSON Scalar.lvclass">)  [unwired: 8 in]
                    }
                    n142 = call "Write Array.vi"("error in (no error)"=w489, "Array"=w490) -> ("error out"=w488:errorcluster, "JSON Array out"=w487:refnum<class "JSON Array.lvclass">)  [unwired: 8 in]
                  }
                  n143 = call "Write Array.vi"("error in (no error)"=w480, "Array"=w481) -> ("error out"=w479:errorcluster, "JSON Array out"=w478:refnum<class "JSON Array.lvclass">)  [unwired: 8 in]
                }
              }
            }
            frame Default {
              n144 = call "Variant Decode.vi"("error in (no error)"=w497, "variant"=w498) -> ("error out"=w503:errorcluster, "Array Dimensions (Reversed)"=w501:i32[], "Variant Data"=w502:T3[])  [unwired: 7 in]
              n145 = call "MultiD Array to JSON.vi"("Treatment of Infinity/NaN"=w499, "error in (no error)"=w503, "Array Dimensions"=w501, "Variant Data"=w502) -> ("error out"=w504:errorcluster, "JSON Array out"=w500:refnum<class "JSON Array.lvclass">)  [unwired: 5 in, 1 out]
            }
          }
        }
        frame "Cluster" {
          n146 = call "Variant Decode.vi"("error in (no error)"=w506, "variant"=w508) -> ("error out"=w507:errorcluster, "Variant Data"=w509:T3[])  [unwired: 7 in, 1 out]
          n147 = for {
            shift-right: [w522] -> w511
            shift-left: refnum<class "JSON Object.lvclass"> refnum ("JSON Object out") -> [w521]
            shift-right: [w519] -> w510
            shift-left: w507 -> [w514]
            tunnel: w509 -> [w518] mode=indexing
            tunnel: w505 -> [w513]
            n148 = call "Handle JSON Text Tag.vi"("Variant Data"=w518) -> ("Variant Data (tag stripped)"=w515:T3)  [unwired: 9 in, 1 out]
            n149 = Unbundle By Name(w515) -> ("Name"=w517:string, "Variant"=w516:variant)
            n150 = call "Variant to JSON.vi"("Treatment of Infinity/NaN"=w513, "error in (no error)"=w514, "Variant"=w516) -> ("error out"=w520:errorcluster, "JSON Value out"=w523:refnum<class "JSON Value.lvclass">)  [unwired: 7 in]
            n151 = call-dynamic "Set Item by name.vi"("error in (no error)"=w520, "Value"=w523, "name"=w517, "JSON Object in"=w521) -> ("error out"=w519:errorcluster, "JSON Object out"=w522:refnum<class "JSON Object.lvclass">)  [unwired: 5 in, 1 out]
          }
        }
        frame "Variant", "LV Variant" {
          n152 = Variant To Data(error in=w525, type=variant, Variant=w526) -> (data=w529:variant, error out=w528:errorcluster)
          n153 = call "Variant to JSON.vi"("Treatment of Infinity/NaN"=w524, "error in (no error)"=w528, "Variant"=w529) -> ("error out"=w530:errorcluster, "JSON Value out"=w531:refnum<class "JSON Value.lvclass">)  [unwired: 7 in]
        }
        frame "Waveform" {
          n154 = Variant To Data(error in=w536, type=waveform(dbl) {"t0"=timestamp(0 s since 1904-01-01), "dt"=1.0, "Y"=[]} ("waveform"), Variant=w537) -> (data=w533:waveform(dbl), error out=w532:errorcluster)
          n155 = call "Set Waveform.vi"("Treatment of Infinity/NaN"=w535, "error in (no error)"=w532, "waveform"=w533) -> ("error out"=w538:errorcluster, "JSON Object out"=w539:refnum<class "JSON Object.lvclass">)  [unwired: 7 in]
        }
        frame "Timestamp" {
          n156 = Variant To Data(error in=w540, type=timestamp(0 s since 1904-01-01), Variant=w544) -> (data=w542:timestamp, error out=w541:errorcluster)
          n157 = call-poly "Set (polymorphic).vi"("error in (no error)"=w541, "Time Stamp"=w542) -> ("error out"=w545:errorcluster, "JSON Scalar out"=w546:refnum<class "JSON Scalar.lvclass">)  [unwired: 8 in]
        }
        frame "Refnum" {
          n158 = call <vilib>:"GetRefnumInfo.vi"("error in (no error)"=w549, "Variant"=w550) -> ("error out"=w553:errorcluster, "ReferenceType"=w551:T4)  [unwired: 6 in, 2 out]
          n159 = case shown="Default" w551 {
            selector: w551 -> [w557 _ _]
            tunnel: [w556 w560 w564] -> w552
            tunnel: w553 -> [w558 w562 w566]
            tunnel: [w555 w559 w565] -> w554
            tunnel: w550 -> [_ w563 w569]
            frame "NotARefnum", "UnknownRefnum" {
              n160 = call <userlib>:"Get Strings from Enum__ogtk.vi"("error in (no error)"=w558, "Enum"=w557) -> ("error out"=w555:errorcluster, "String Value"=w556:string)  [unwired: 6 in, 2 out]
            }
            frame "Visa", "IVI", "UserDefinedRefnumTag" {
              n161 = Variant To Data(error in=w562, type="", Variant=w563) -> (data=w560:string, error out=w559:errorcluster)
            }
            frame Default {
              n162 = Variant To Flattened String(Variant=w569) -> (data string=w568:string)  [unwired: 1 out]
              n163 = Type Cast(type=0, x=w568) -> (*(type *) &x=w567:i32)
              n164 = Format Into String(error in=w566, w567) -> (resulting string=w564:string, error out=w565:errorcluster)  [unwired: 2 in]
            }
          }
          n165 = call-poly "Set (polymorphic).vi"("error in (no error)"=w554, "String"=w552) -> ("error out"=w547:errorcluster, "JSON Scalar out"=w548:refnum<class "JSON Scalar.lvclass">)  [unwired: 8 in]
        }
        frame "LabVIEW Class Instance" {
          w575 = refnum<class "JSON Value.lvclass"> refnum  # JSON Value
          n166 = Variant To Data(error in=w579, type=refnum<class> refnum ("LabVIEW Object"), Variant=w580) -> (data=w576:refnum<class>, error out=w571:errorcluster)
          n167 = To More Specific Class(target class=w575, reference=w576, error in=w571) -> (error out=w577:errorcluster)  [unwired: 1 out]
          n168 = case shown="No Error" w577 {
            selector: w577 -> [w581 _]
            tunnel: w576 -> [w585 w590]
            tunnel: w575 -> [w584 _]
            tunnel: [w583 w588] -> w574
            tunnel: [w582 w586] -> w572
            frame No Error {
              # "A JSON Value already, so just\nuse it"
              n169 = To More Specific Class(target class=w584, reference=w585, error in=w581) -> (specific class reference=w583:refnum<class "JSON Value.lvclass">, error out=w582:errorcluster)
            }
            frame Error {
              # "For lack of a better thing to do,\nflatten to string."
              n170 = Flatten To String(anything=w590) -> (data string=w589:string, error out=w587:errorcluster)  [unwired: 3 in, 1 out]
              n171 = call "Set String.vi"("error in (no error)"=w587, "String"=w589) -> ("error out"=w586:errorcluster, "JSON Scalar out"=w588:refnum<class "JSON Scalar.lvclass">)  [unwired: 8 in]
            }
          }
          n172 = Merge Errors(w571, w572) -> (w573:errorcluster)
        }
        frame Default {
          # "For lack of a better thing to do,\nflatten to string."
          n173 = Variant To Flattened String(Variant=w592) -> (data string=w591:string)  [unwired: 1 out]
          n174 = call "Set String.vi"("error in (no error)"=w593, "String"=w591) -> ("error out"=w594:errorcluster, "JSON Scalar out"=w595:refnum<class "JSON Scalar.lvclass">)  [unwired: 8 in]
        }
      }
    }
    frame Error {
    }
  }
  "error out" <- w4
  "JSON Value out" <- w3
